vi "LabJack U3 Settings Dialog.vi"(8 "error in (no error)":errorcluster, 11 "U3 Module Config in":T2) -> (0 "error out":errorcluster, 1 "Cancelled?":bool=TRUE, 2 "UI Refresh Needed?":bool, 3 "U3 Module Config out":T2)   [LabVIEW 2018, in "LabJack U3 Module.lvlib"]
doc: "Dialog for selecting user specified settings."
uses:
  LabJack U3 Module.lvlib
  controls/LabJack U3 Module Config Cluster.ctl
  <vilib>/Utility/miscctls.llb/LVPoint32TypeDef.ctl
  controls/LabJack U3 Settings Dialog.ctl
  Tag VIs/Tag FGV Operation Enum.ctl
  Shared Variables/Simple Alarm Values Cluster.ctl
  Shared Variables/Dynamic Shared Variables.lvlib
panel:
  in  "Settings Dialog":T1 {"Input Channel Tag Name" items=["AI0", "AI1", "AI2", "AI3", "AI4", "AI5", "AI6", "AI7"]; "LoLo" max=8.0 step=1.0}
  in  "Cancel Button":bool
  in  "OK Button":bool
  # "Non visible portion of dialog (needed for connector pane)."
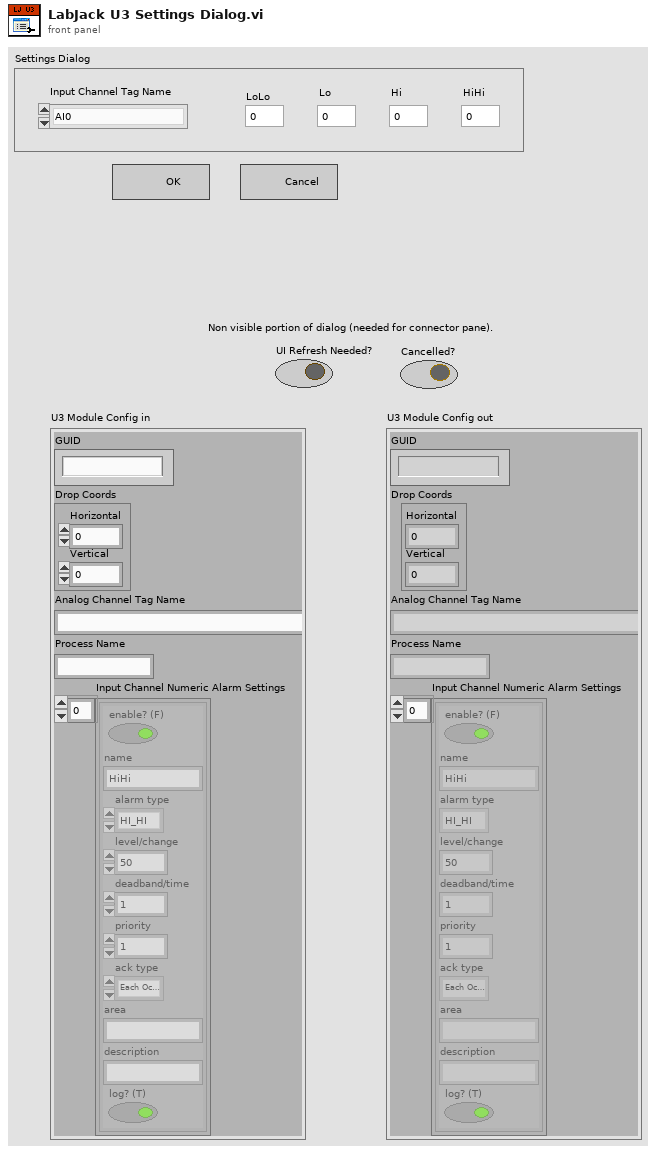
[diagram p1: front panel]
types:
  T1 = typedef "LabJack U3 Module.lvlib/LabJack U3 Settings Dialog.ctl" = cluster{"LoLo":dbl, "Lo":dbl, "Hi":dbl, "HiHi":dbl, "Input Channel Tag Name":u16}
  T2 = typedef "LabJack U3 Module.lvlib/LabJack U3 Module Config Cluster.ctl" = cluster{"GUID":string, "Drop Coords":T3, "Analog Channel Tag Name ":string, "Process Name":string, "Input Channel Numeric Alarm Settings":cluster{"enable? (F)":bool, "name":string, "alarm type":enum16{"HI_HI", "HI", "LO", "LO_LO"}, "level/change":dbl, "deadband/time":dbl, "priority":u32, "ack type":enum16{"Auto", "User", "None", "Each Occurrence"}, "area":string, "description":string, "log? (T)":bool}[]}
  T3 = typedef "LVPoint32TypeDef.ctl" = cluster{"Horizontal":i32, "Vertical":i32}
  T4 = typedef "Tag FGV Operation Enum.ctl" = enum16{"Init", "Set Notification Queue", "Create Tag", "Write Tag (Numeric)", "Write Tag (Boolean)", "Read All Tags", "Read One Tag", "Delete Tag Category", "Set Alarm Parameters (Numeric)", "Set Alarm Parameters (Boolean)", "Enable All Alarms", "Disable All Alarms", "Delete All Tags", "Read Alarms", "Ack Alarm"}
  T5 = typedef "Dynamic Shared Variables.lvlib/Simple Alarm Values Cluster.ctl" = cluster{"tag name":string, "HiHi":dbl, "Hi":dbl, "Lo":dbl, "LoLo":dbl}
  T6 = cluster{"enable? (F)":bool, "name":string, "alarm type":enum16{"HI_HI", "HI", "LO", "LO_LO"}, "level/change":dbl, "deadband/time":dbl, "priority":u32, "ack type":enum16{"Auto", "User", "None", "Each Occurrence"}, "area":string, "description":string, "log? (T)":bool}[]
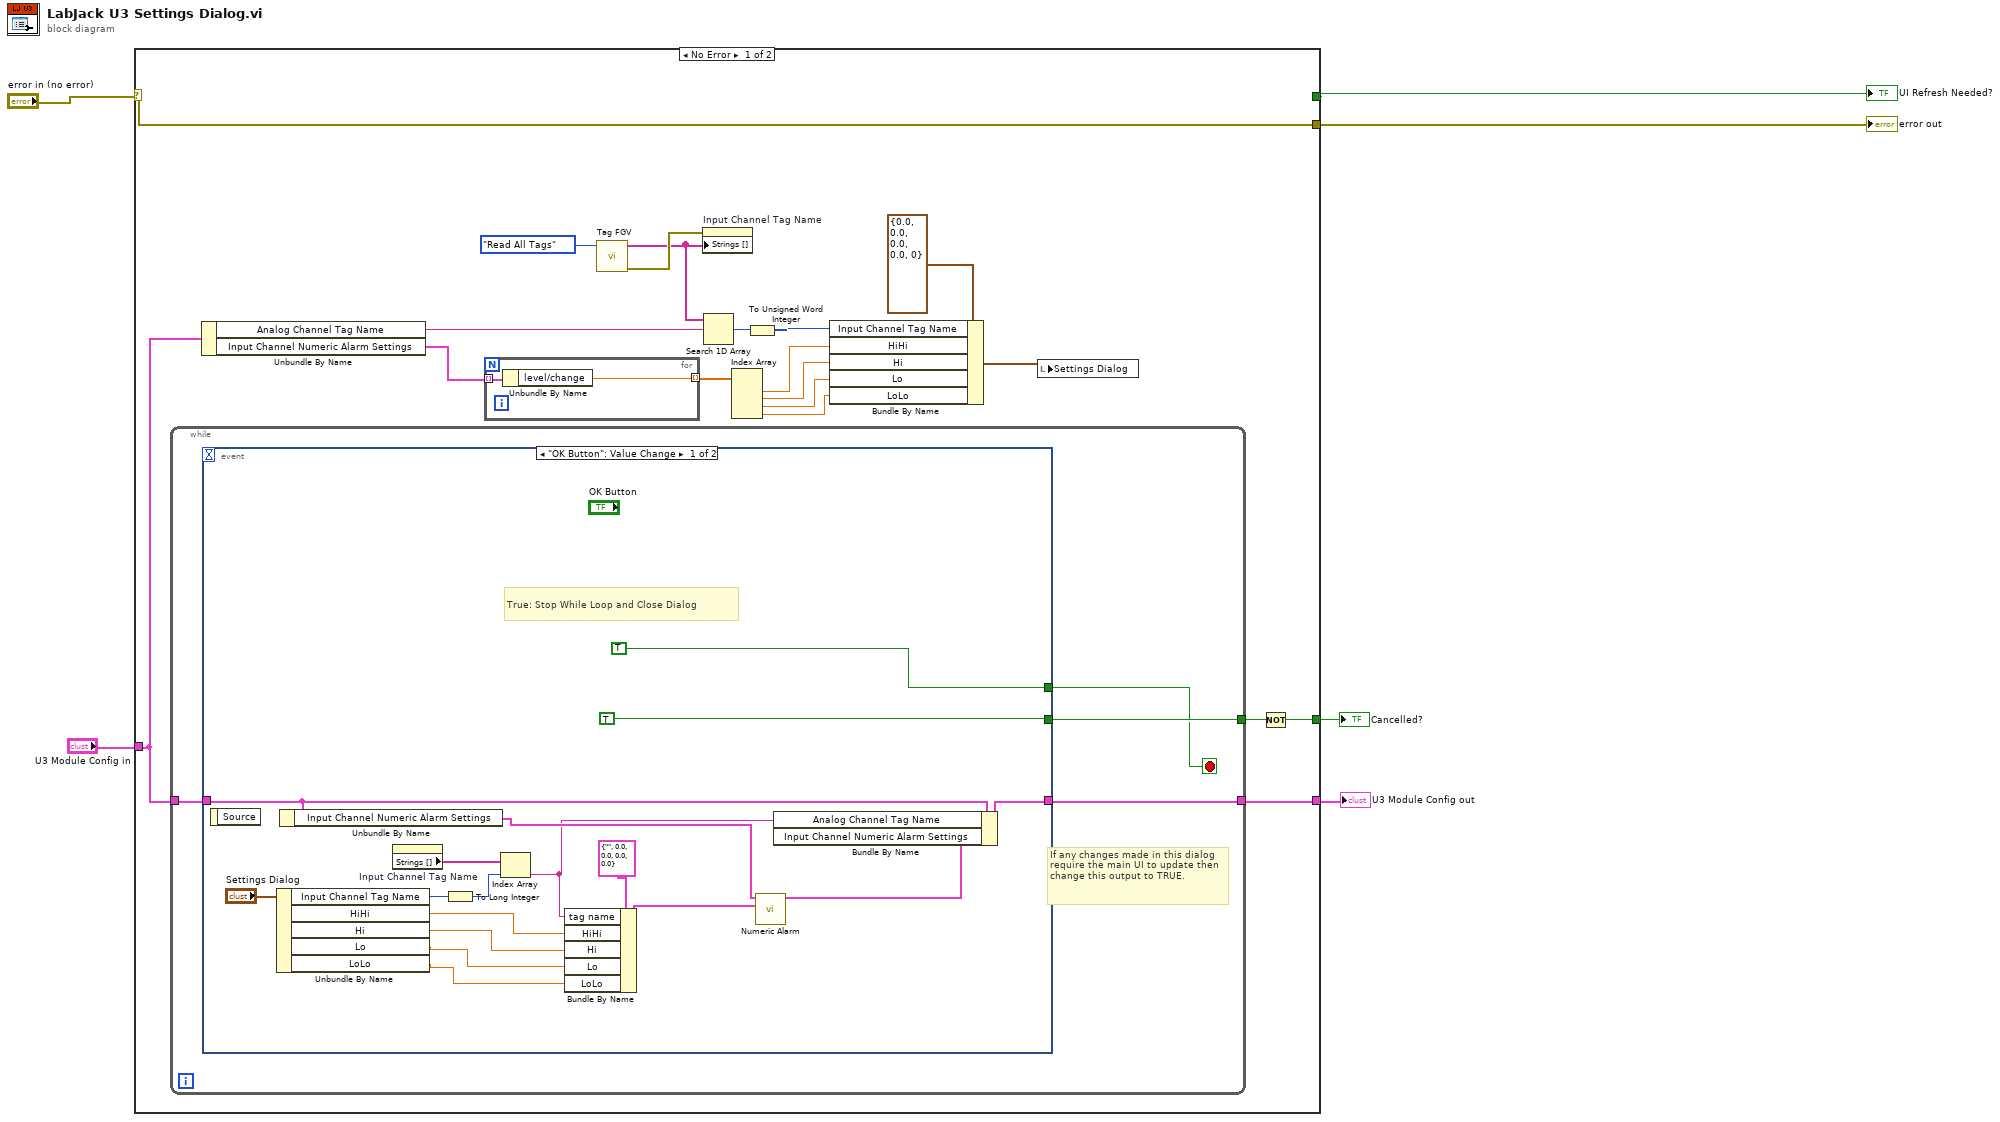
[diagram p0: block diagram]
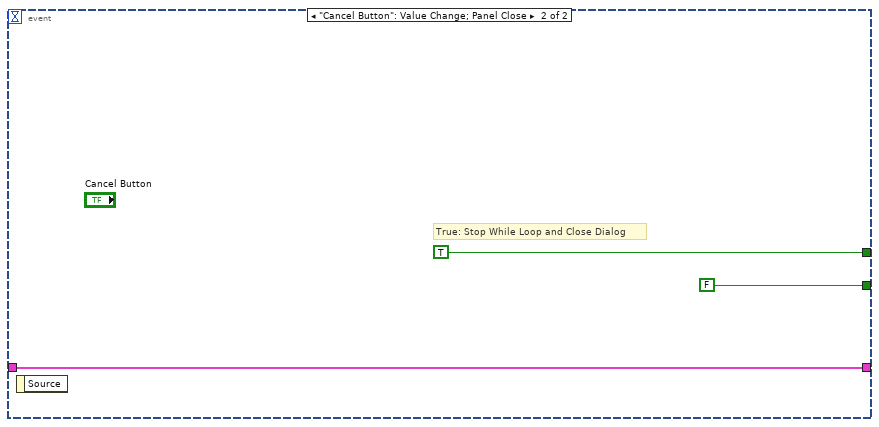
[diagram p2: hidden frame]
diagram:
  n1 = case shown="No Error" "error in (no error)" {
    selector: "error in (no error)" -> [w26 w55]
    tunnel: [w26 w55] -> w6
    tunnel: "U3 Module Config in" -> [w23 w54]
    tunnel: [w24 w54] -> w1
    tunnel: [FALSE ("UI Refresh Needed?") _] -> w4
    tunnel: [w21 TRUE ("UI Refresh Needed?")] -> w3
    frame No Error {
      n2 = while {
        tunnel: [w32] -> w22
        tunnel: [w29] -> w24
        tunnel: w23 -> [w31]
        stop <- w30 stop-if-true
        # "If any changes made in this dialog require the main UI to update then change this output to TRUE."
        n3 = event shown="[0] \"OK Button\": Value Change" {
          selector: _ -> [_ _]
          dyn-events: _ -> [_ _]
          timeout: _ -> [_ _]
          tunnel: w31 -> [w42 w52]
          tunnel: [TRUE ("UI Refresh Needed?") FALSE ("UI Refresh Needed?")] -> w32
          tunnel: [TRUE TRUE] -> w30
          tunnel: [w46 w52] -> w29
          event "OK Button": Value Change {
            # "True: Stop While Loop and Close Dialog"
            n4 = event-data() -> ()  [unwired: 1 in, 1 out]
            n5 = Unbundle By Name("Settings Dialog") -> ("Input Channel Tag Name"=w44:u16, "HiHi"=w38:dbl, "Hi"=w37:dbl, "Lo"=w36:dbl, "LoLo"=w35:dbl)
            n6 = Unbundle By Name(w42) -> ("Input Channel Numeric Alarm Settings"=w41:T6)
            n7 = property on="Input Channel Tag Name" class="Ring (strict)"() -> ("Strings []"=w45:string[])  [unwired: 2 in, 2 out]
            n8 = To Long Integer(number=w44) -> (32bit integer=w43:i32)
            n9 = Index Array(array=w45, index=w43) -> (element=w39:string)
            n10 = Bundle By Name(cluster=T5 {"tag name"="", "HiHi"=0.0, "Hi"=0.0, "Lo"=0.0, "LoLo"=0.0} ("Simple Alarm Values"), "tag name"=w39, "HiHi"=w38, "Hi"=w37, "Lo"=w36, "LoLo"=w35) -> (w33:T5)
            n11 = call "Numeric Alarm.vi"("Simple Alarm Values"=w33, "Alarms in"=w41) -> ("Alarms out"=w40:T6)  [unwired: 9 in]
            n12 = Bundle By Name(cluster=w42, "Analog Channel Tag Name"=w39, "Input Channel Numeric Alarm Settings"=w40) -> (w46:T2)
          }
          event "Cancel Button": Value Change; Panel Close {
            # "True: Stop While Loop and Close Dialog"
            n13 = event-data() -> ()  [unwired: 1 in, 1 out]
          }
        }
      }
      n14 = Unbundle By Name(w23) -> ("Analog Channel Tag Name"=w18:string, "Input Channel Numeric Alarm Settings"=w16:T6)
      n15 = for {
        tunnel: w16 -> [w28] mode=indexing
        tunnel: [w27] -> w12 mode=indexing
        n16 = Unbundle By Name(w28) -> ("level/change"=w27:dbl)
      }
      n17 = call "Tag FGV.vi"("Operation"=Tag_FGV_Operation_Enum."Read All Tags") -> ("error out"=w20:errorcluster, "Tag Names"=w7:string[])  [unwired: 5 in, 4 out]
      n18 = property on="Input Channel Tag Name" class="Ring (strict)"(error in=w20, "Strings []"=w7) -> ()  [unwired: 1 in, 2 out]
      n19 = Search 1D Array(1D array=w7, element=w18) -> (index of element=w17:i32)  [unwired: 1 in]
      n20 = Index Array(array=w12) -> (element #1=w11:dbl, element #2=w10:dbl, element #3=w9:dbl, element #4=w8:dbl)  [unwired: 4 in]
      n21 = To Unsigned Word Integer(number=w17) -> (unsigned 16bit integer=w14:u16)
      n22 = Bundle By Name(cluster=T1 {"LoLo"=0.0, "Lo"=0.0, "Hi"=0.0, "HiHi"=0.0, "Input Channel Tag Name"=0} ("Settings Dialog"), "Input Channel Tag Name"=w14, "HiHi"=w11, "Hi"=w10, "Lo"=w9, "LoLo"=w8) -> (w13:T1)
      n23 = local write "Settings Dialog"(w13) -> ()
      n24 = Not(x=w22) -> (.not. x?=w21:bool)
    }
    frame Error {
    }
  }
  "UI Refresh Needed?" <- w4
  "error out" <- w6
  "U3 Module Config out" <- w1
  "Cancelled?" <- w3
